vi "Decode Trigger Time.vi"(8 "Comm_order":i16, 10 "Trigger_time string":string) -> (3 "Trigger Time":T1)   [LabVIEW 2013, in "LeCroy Wave Series.lvlib"]
doc: "Decode trigger time from data string that is readout from the descriptor block field."
uses:
  <instrlib>/LeCroy Wave Series/LeCroy Wave Series.lvlib
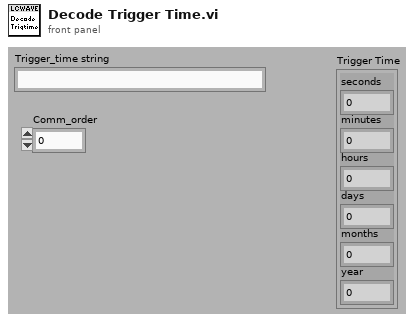
[diagram p1: front panel]
types:
  T1 = cluster{"seconds":dbl, "minutes":u8, "hours":u8, "days":u8, "months":u8, "year":u16}
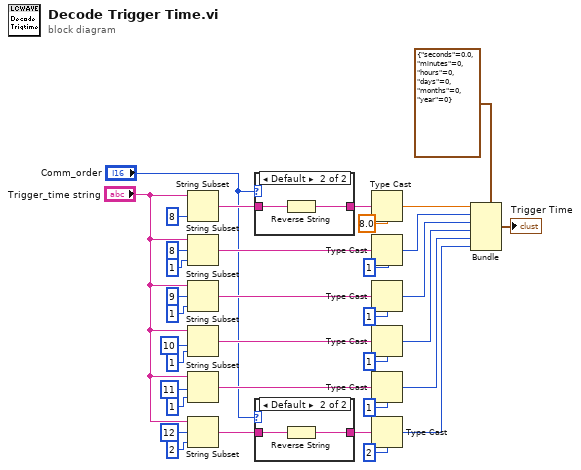
[diagram p0: block diagram]
diagram:
  n1 = String Subset(string="Trigger_time string", length (rest)=8 ("length (rest)")) -> (substring=w4:string)  [unwired: 1 in]
  n2 = String Subset(string="Trigger_time string", offset (0)=8, length (rest)=1 ("length (rest)")) -> (substring=w20:string)
  n3 = String Subset(string="Trigger_time string", offset (0)=9, length (rest)=1 ("length (rest)")) -> (substring=w21:string)
  n4 = String Subset(string="Trigger_time string", offset (0)=10, length (rest)=1 ("length (rest)")) -> (substring=w22:string)
  n5 = String Subset(string="Trigger_time string", offset (0)=11, length (rest)=1 ("length (rest)")) -> (substring=w23:string)
  n6 = String Subset(string="Trigger_time string", offset (0)=12, length (rest)=2 ("length (rest)")) -> (substring=w1:string)
  n7 = case shown="Default" "Comm_order" {
    tunnel: [w36 w37] -> w5
    tunnel: w4 -> [w36 w38]
    frame 0 {
    }
    frame Default {
      n8 = Reverse String(1:w38) -> (0:w37:string)
    }
  }
  n9 = case shown="Default" "Comm_order" {
    tunnel: [w39 w40] -> w3
    tunnel: w1 -> [w39 w41]
    frame 0 {
    }
    frame Default {
      n10 = Reverse String(1:w41) -> (0:w40:string)
    }
  }
  n11 = Type Cast(type=8.0 ("length (rest)"), x=w5) -> (*(type *) &x=w13:dbl)
  n12 = Type Cast(type=u8 1 ("length (rest)"), x=w20) -> (*(type *) &x=w12:u8)
  n13 = Type Cast(type=u8 1 ("length (rest)"), x=w21) -> (*(type *) &x=w11:u8)
  n14 = Type Cast(type=u8 1 ("length (rest)"), x=w22) -> (*(type *) &x=w10:u8)
  n15 = Type Cast(type=u8 1 ("length (rest)"), x=w23) -> (*(type *) &x=w9:u8)
  n16 = Type Cast(type=u16 2 ("length (rest)"), x=w3) -> (*(type *) &x=w8:u16)
  n17 = Bundle(cluster=T1 {"seconds"=0.0, "minutes"=0, "hours"=0, "days"=0, "months"=0, "year"=0}, "seconds"=w13, "minutes"=w12, "hours"=w11, "days"=w10, "months"=w9, "year"=w8) -> (→"Trigger Time":T1)
